vi "TSDiscovery Object--constant.vi"() -> (3 "TSDiscovery.lvclass":refnum<class "TSDiscovery.lvclass">)   [LabVIEW 2025]
doc: "Return an object of TSDiscovery.lvclass."
uses:
  TSDiscovery/TSDiscovery.lvclass
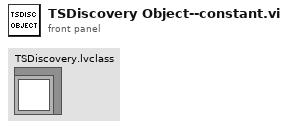
[diagram p1: front panel]
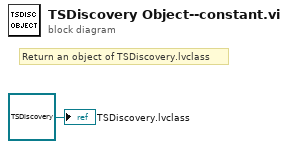
[diagram p0: block diagram]
diagram:
  # "Return an object of TSDiscovery.lvclass"
  "TSDiscovery.lvclass" <- refnum<class "TSDiscovery.lvclass"> refnum ("TSDiscovery.lvclass")
